vi "Finalize Configuration.vi"(8 "error in (no error)":errorcluster, 11 "config data":T1) -> (0 "error out":errorcluster, 3 "file json":string)   [LabVIEW 2017, in "DSF Core.lvlib" / "Configuration Session.lvclass"]
uses:
  Configuration Session.lvclass
  Internal DSF Configuration.ctl
  Typedefs/DSF Version Info.ctl
  Internal DSF Plugin with ID.ctl
  Internal DSF Plugin Info.ctl
  Typedefs/DSF Timing Info.ctl
  Typedefs/DSF Engine Plugin Thread Configuration.ctl
  Typedefs/DSF Settings Info.ctl
  Internal DSF Group with ID.ctl
  Internal DSF Group Info.ctl
  Internal DSF Transfer with ID.ctl
  Internal DSF Transfer Info.ctl
  Internal DSF Channel with ID.ctl
  Internal DSF Channel Info.ctl
  Internal DSF Settings with ID.ctl
  Internal DSF Settings Info.ctl
  Typedefs/DSF Engine Framework Configuration.ctl
  Typedefs/DSF Engine Plugin Configuration.ctl
  Typedefs/DSF Engine Transfer Group Configuration.ctl
  Typedefs/DSF Direction.ctl
  Typedefs/DSF Engine Transfer Configuration.ctl
  Typedefs/DSF Byte Order.ctl
  Typedefs/DSF Engine Channel Configuration.ctl
  Typedefs/DSF Data Type.ctl
  Typedefs/DSF Timeout Behavior.ctl
  DSF Core.lvlib
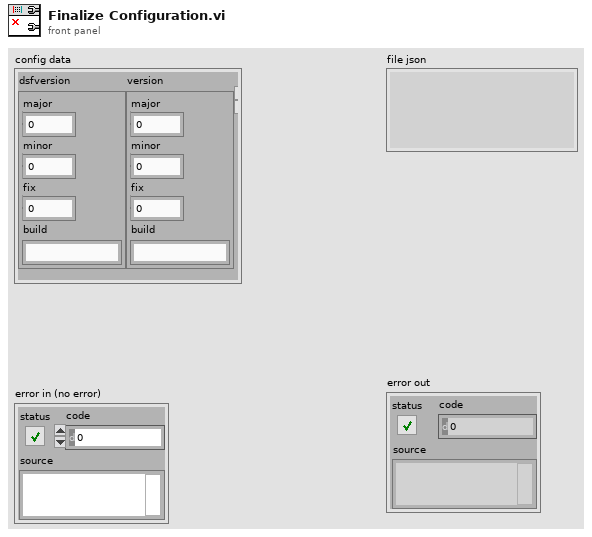
[diagram p1: front panel]
types:
  T1 = typedef "DSF Core.lvlib/Configuration Session.lvclass/Internal DSF Configuration.ctl" = cluster{"dsfversion":T2, "version":T2, "plugins":T3[], "groups":T8[], "transfers":T10[], "channels":T12[], "settings":T14[], "framework configuration":T16}
  T2 = typedef "DSF Core.lvlib/DSF Version Info.ctl" = cluster{"major":u32, "minor":u32, "fix":u32, "build":string}
  T3 = typedef "DSF Core.lvlib/Configuration Session.lvclass/Internal DSF Plugin with ID.ctl" = cluster{"id":string, "values":T4}
  T4 = typedef "DSF Core.lvlib/Configuration Session.lvclass/Internal DSF Plugin Info.ctl" = cluster{"components":string[], "timing":T5, "group ids":string[], "settings id":string, "threads":T6[]}
  T5 = typedef "DSF Core.lvlib/DSF Timing Info.ctl" = cluster{"priority":u64, "decimation":u64, "offset":u64}
  T6 = typedef "DSF Core.lvlib/DSF Engine Plugin Thread Configuration.ctl" = cluster{"buffer converter settings":T7, "transceiver settings":T7, "custom settings":T7, "processor":i32, "priority offset":i16}
  T7 = typedef "DSF Core.lvlib/DSF Settings Info.ctl" = cluster{"key":string, "value":string}[]
  T8 = typedef "DSF Core.lvlib/Configuration Session.lvclass/Internal DSF Group with ID.ctl" = cluster{"id":string, "values":T9}
  T9 = typedef "DSF Core.lvlib/Configuration Session.lvclass/Internal DSF Group Info.ctl" = cluster{"direction":i32, "timing":T5, "transfer ids":string[], "settings id":string, "thread":i32, "timeout behavior":u8}
  T10 = typedef "DSF Core.lvlib/Configuration Session.lvclass/Internal DSF Transfer with ID.ctl" = cluster{"id":string, "values":T11}
  T11 = typedef "DSF Core.lvlib/Configuration Session.lvclass/Internal DSF Transfer Info.ctl" = cluster{"byte order":i32, "channel ids":string[], "settings id":string}
  T12 = typedef "DSF Core.lvlib/Configuration Session.lvclass/Internal DSF Channel with ID.ctl" = cluster{"id":string, "values":T13}
  T13 = typedef "DSF Core.lvlib/Configuration Session.lvclass/Internal DSF Channel Info.ctl" = cluster{"string buffer offset":u64, "string data type":i32, "engine data type":i32, "settings id":string, "units":string}
  T14 = typedef "DSF Core.lvlib/Configuration Session.lvclass/Internal DSF Settings with ID.ctl" = cluster{"id":string, "values":T15}
  T15 = typedef "DSF Core.lvlib/Configuration Session.lvclass/Internal DSF Settings Info.ctl" = cluster{"key":string, "value":string}[]
  T16 = typedef "DSF Core.lvlib/DSF Engine Framework Configuration.ctl" = cluster{"Plugins":T17[]}
  T17 = typedef "DSF Core.lvlib/DSF Engine Plugin Configuration.ctl" = cluster{"name":string, "components":string[], "cycle timing":T5, "threads":T6[], "Transfer Groups":T18[], "settings":T7}
  T18 = typedef "DSF Core.lvlib/DSF Engine Transfer Group Configuration.ctl" = cluster{"name":string, "direction":T19, "cycle timing":T5, "thread index":i32, "settings":T7, "Transfers":T20[], "timeout behavior":T24}
  T19 = typedef "DSF Core.lvlib/DSF Direction.ctl" = enum8{"Tx", "Rx"}
  T20 = typedef "DSF Core.lvlib/DSF Engine Transfer Configuration.ctl" = cluster{"name":string, "byte order":T21, "settings":T7, "channels":T22[]}
  T21 = typedef "DSF Core.lvlib/DSF Byte Order.ctl" = enum8{"big-endian", "little-endian"}
  T22 = typedef "DSF Core.lvlib/DSF Engine Channel Configuration.ctl" = cluster{"string offset":u64, "string data type":T23, "engine data type":T23, "name":string, "settings":T7, "units":string}
  T23 = typedef "DSF Core.lvlib/DSF Data Type.ctl" = enum8{"Bool", "SGL", "DBL", "I8", "I16", "I32", "I64", "U8", "U16", "U32", "U64"}
  T24 = typedef "DSF Core.lvlib/DSF Timeout Behavior.ctl" = enum8{"Increment Late Count", "Throw Error"}
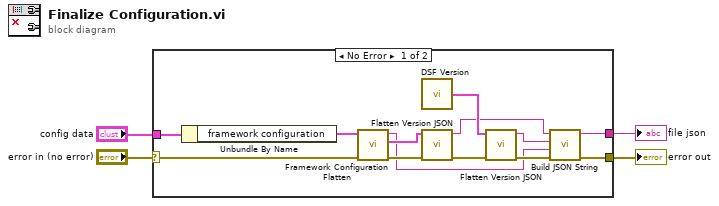
[diagram p0: block diagram]
diagram:
  n1 = case shown="No Error" "error in (no error)" {
    selector: "error in (no error)" -> [w5 w18]
    tunnel: "config data" -> [w17 _]
    tunnel: [w10 w18] -> w3
    tunnel: [w9 _] -> w2
    frame No Error {
      n2 = Unbundle By Name(w17) -> ("framework configuration"=w16:T16)
      n3 = call "Framework Configuration Flatten.vi"("error in (no error)"=w5, "framework configuration"=w16) -> ("error out"=w15:errorcluster, "json version"=w14:T2, "dsf configuration json"=w6:string)  [unwired: 7 in]
      n4 = call "DSF Version.vi"() -> ("dsf version"=w12:T2)  [unwired: 1 in]
      n5 = call "Flatten Version JSON.vi"("error in (no error)"=w15, "version"=w14) -> ("error out"=w13:errorcluster, "version json"=w7:string)  [unwired: 8 in]
      n6 = call "Flatten Version JSON.vi"("error in (no error)"=w13, "version"=w12) -> ("error out"=w11:errorcluster, "version json"=w8:string)  [unwired: 8 in]
      n7 = call "Build JSON String.vi"("error in (no error)"=w11, "dsf configuration substring"=w6, "dsf version substring"=w8, "json version substring"=w7) -> ("error out"=w10:errorcluster, "string"=w9:string)  [unwired: 6 in]
    }
    frame Error {
    }
  }
  "file json" <- w2
  "error out" <- w3
